vi "1.2 - Building red and IR LED drivers-2.vi"() -> ()   [LabVIEW 2017]
uses:
  <vilib>/measure/NI_MABase.lvlib
panel:
  out "data":dynamicdata(graph)
  out "signal out":waveform(dbl)
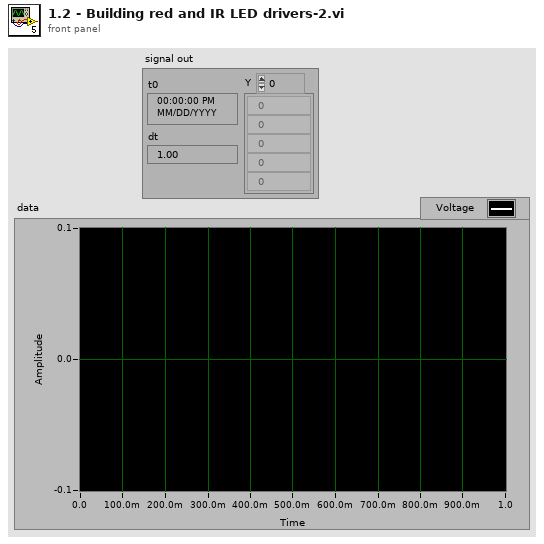
[diagram p1: front panel]
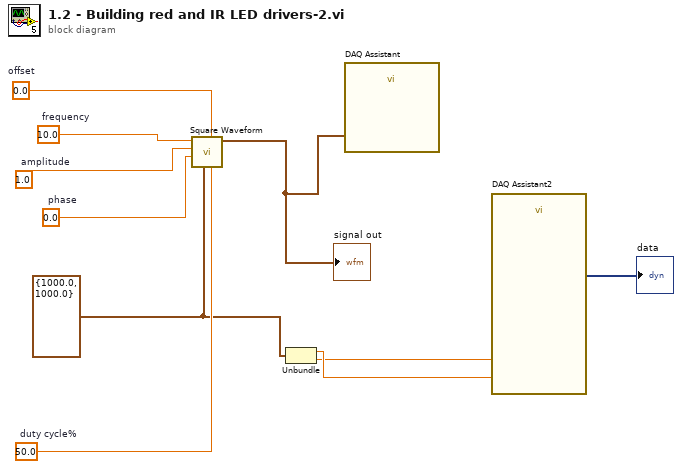
[diagram p0: block diagram]
diagram:
  w5 = cluster{"Fs":dbl, "#s":dbl} {"Fs"=1000.0, "#s"=1000.0} ("sampling info")
  w6 = 50.0  # duty cycle%
  w8 = 1.0  # amplitude
  w7 = 0.0  # phase
  w9 = 10.0  # frequency
  w10 = 0.0  # offset
  n1 = call <vilib>:"Square Waveform.vi"("duty cycle (%)"=w6, "offset"=w10, "sampling info"=w5, "phase"=w7, "amplitude"=w8, "frequency"=w9) -> ("signal out"=w4:waveform(dbl))  [unwired: 4 in, 1 out]
  "signal out" <- w4
  n2 = Unbundle(w5) -> ("Fs"=w3:dbl, "#s"=w2:dbl)
  n3 = call "DAQ Assistant"("data"=w4) -> ()  [unwired: 17 in, 2 out]
  n4 = call "DAQ Assistant2"("rate"=w3, "number of samples"=w2) -> ("data"=→"data":dynamicdata)  [unwired: 15 in, 2 out]
